vi "Get StationGlobals Prop.vi"(8 "error in (no error)":errorcluster, 11 "TSEngine in":refnum<class "Engine.lvclass">) -> (0 "error out":errorcluster, 2 "StationGlobals":T1, 3 "TSEngine out":refnum<class "Engine.lvclass">)   [LabVIEW 2019, in "HTS.lvlib" / "Engine.lvclass"]
uses:
  Engine.lvclass
  Variable Container Type.ctl
  VariableContainer/VariableContainer.lvclass
  VariableContainer/Typedefs/Session Handle.ctl
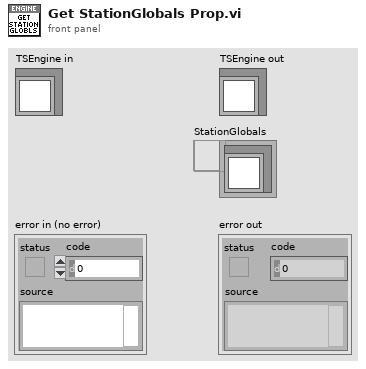
[diagram p1: front panel]
types:
  T1 = typedef "HTS.lvlib/VariableContainer.lvclass/Session Handle.ctl" = refnum<data-value>
  T2 = typedef "HTS.lvlib/Engine.lvclass/Variable Container Type.ctl" = enum16{"StationGlobals", "TemporaryGlobals", "NewPropertyObject"}
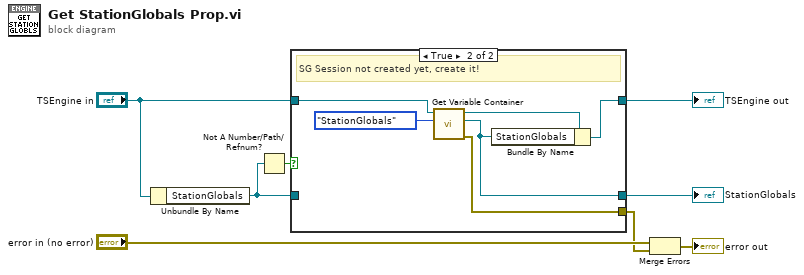
[diagram p0: block diagram]
diagram:
  n1 = Unbundle By Name("TSEngine in") -> ("StationGlobals"=w6:T1)
  n2 = Not A Number/Path/Refnum?(number/path/refnum=w6) -> (NaN/Path/Refnum?=w7:bool)
  n3 = case shown="True" w7 {
    tunnel: w6 -> [w10 _]
    tunnel: [w10 w12] -> w5
    tunnel: "TSEngine in" -> [w9 w15]
    tunnel: [w9 w16] -> w2
    tunnel: [_ w11] -> w1
    frame False {
      # "SG session already created, return existing session."
    }
    frame True {
      # "SG Session not created yet, create it!"
      n4 = call "Get Variable Container.vi"("Type"=Variable_Container_Type."StationGlobals", "TSEngine in"=w15) -> ("error out"=w11:errorcluster, "VariableContainer"=w12:T1, "TSEngine out"=w13:refnum<class "Engine.lvclass">)  [unwired: 7 in]
      n5 = Bundle By Name(cluster=w13, "StationGlobals"=w12) -> (w16:refnum<class "Engine.lvclass">)
    }
  }
  "TSEngine out" <- w2
  "StationGlobals" <- w5
  n6 = Merge Errors("error in (no error)", w1) -> (→"error out":errorcluster)
